vi "FGV_tcpConnectionID.vi"(7 "function":enum16{"read", "write"}(ring)=enum."write", 8 "error in (no error)":errorcluster, 10 "connection ID":refnum<k5>) -> (0 "error out":errorcluster, 2 "connection ID out":refnum<k5>)   [LabVIEW 2018, in "TcpServer.lvclass"]
doc: "FGV to store the tcp connection ID to be shared between the read tcp loop and the sender loop, inside of Tcp Server subVI."
uses:
  TcpServer.lvclass
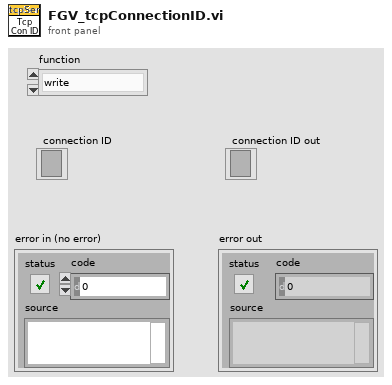
[diagram p1: front panel]
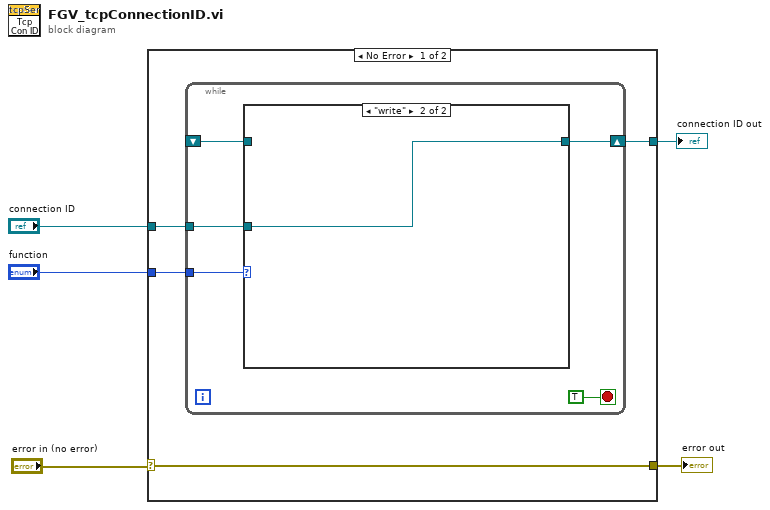
[diagram p0: block diagram]
diagram:
  n1 = case shown="No Error" "error in (no error)" {
    selector: "error in (no error)" -> [w6 w18]
    tunnel: "function" -> [w9 _]
    tunnel: "connection ID" -> [w8 w17]
    tunnel: [w7 w17] -> w3
    tunnel: [w6 w18] -> w1
    frame No Error {
      n2 = while {
        tunnel: w9 -> [w13]
        tunnel: w8 -> [w12]
        shift-right: [w11] -> w7
        shift-left: _ -> [w10]
        stop <- TRUE stop-if-true
        n3 = case shown="\"write\"" w13 {
          tunnel: w12 -> [_ w16]
          tunnel: [w15 w16] -> w11
          tunnel: w10 -> [w15 _]
          frame "read", Default {
          }
          frame "write" {
          }
        }
      }
    }
    frame Error {
    }
  }
  "connection ID out" <- w3
  "error out" <- w1
